vi "Open Screenpop.vi"(8 "error in (no error)":errorcluster, 10 "Open?":bool, 11 "SR Number":i32) -> (0 "error out":errorcluster)   [LabVIEW 2018]
uses:
  <vilib>/Platform/browser.llb/Open URL in Default Browser (string).vi
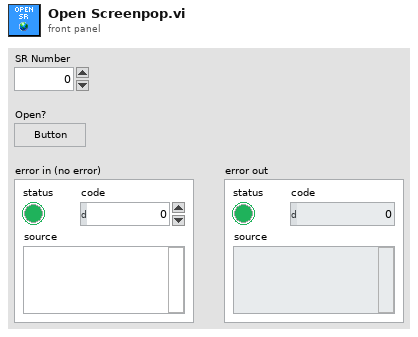
[diagram p1: front panel]
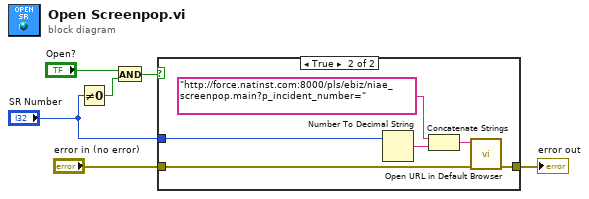
[diagram p0: block diagram]
diagram:
  n1 = Not Equal To 0?(x="SR Number") -> (x != 0?=w2:bool)
  n2 = And(x="Open?", y=w2) -> (x .and. y?=w4:bool)
  n3 = case shown="True" w4 {
    tunnel: "error in (no error)" -> [w7 w13]
    tunnel: [w7 w12] -> w5
    tunnel: "SR Number" -> [_ w8]
    frame False {
    }
    frame True {
      n4 = Number To Decimal String(number=w8) -> (decimal integer string=w11:string)  [unwired: 1 in]
      n5 = Concatenate Strings("http://force.natinst.com:8000/pls/ebiz/niae_screenpop.main?p_incident_number=" ("string"), w11) -> (w9:string)
      n6 = call-poly <vilib>:"Open URL in Default Browser.vi"("error in (no error)"=w13, "URL"=w9) -> ("error out"=w12:errorcluster)  [unwired: 4 in, 1 out]
    }
  }
  "error out" <- w5
